vi "is_finished.vi"(8 "error in (no error)":errorcluster, 11 "ImagingModeDL090130Frame in":refnum<class "ImagingModeDL090130Frame.lvclass">=refnum) -> (0 "error out":errorcluster, 2 "finished?":bool[](array[boolean]), 3 "ImagingModeDL090130Frame out":refnum<class "ImagingModeDL090130Frame.lvclass">)   [LabVIEW 2010, in "ImagingModeDL090130Frame.lvclass"]
uses:
  ImagingModeDL090130Frame.lvclass
  ImagingModeDL090130Frame.lvclass/ImagingModeDL090130Frame.ctl
panel:
  # "element 0: is sweep finished?\nelement 1: frame finished?\nelement 2: consecutive scanning done?"
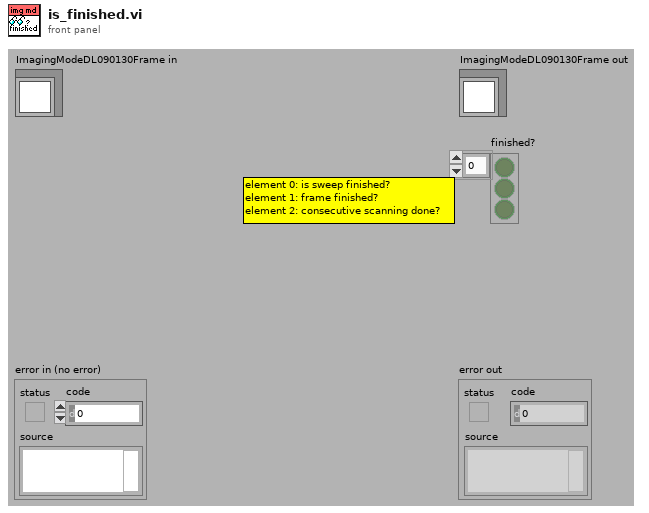
[diagram p1: front panel]
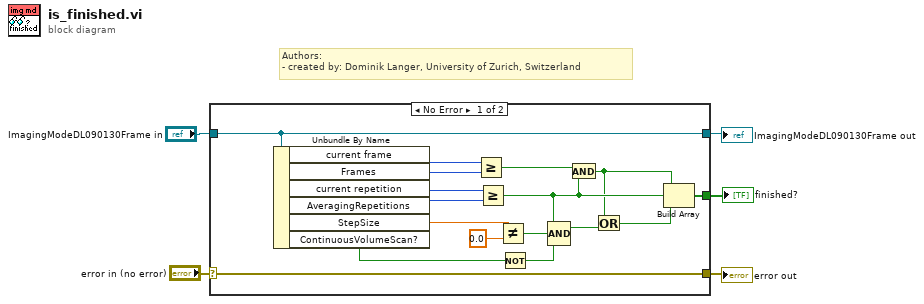
[diagram p0: block diagram]
diagram:
  # "Authors: \n- created by: Dominik Langer, University of Zurich, Switzerland"
  n1 = case shown="No Error" "error in (no error)" {
    selector: "error in (no error)" -> [w13 w24]
    tunnel: [w13 w24] -> w4
    tunnel: [w22 w23] -> w2
    tunnel: "ImagingModeDL090130Frame in" -> [w22 w23]
    tunnel: [w14 _] -> w1
    frame No Error {
      n2 = Unbundle By Name(w22) -> ("current frame"=w21:i32, "Frames"=w20:i32, "current repetition"=w19:i32, "AveragingRepetitions"=w18:i32, "StepSize"=w12:dbl[unit], "ContinuousVolumeScan?"=w8:bool)
      n3 = Greater Or Equal?(x=w21, y=w20) -> (x >= y?=w16:bool)
      n4 = Greater Or Equal?(x=w19, y=w18) -> (x >= y?=w15:bool)
      n5 = Not Equal?(x=w12, y=dbl[unit] 0.0) -> (x != y?=w10:bool)
      n6 = Not(x=w8) -> (.not. x?=w7:bool)
      n7 = Compound Arithmetic op=AND(w15, w10, w7) -> (w17:bool)
      n8 = And(x=w16, y=w15) -> (x .and. y?=w9:bool)
      n9 = Or(x=w9, y=w17) -> (x .or. y?=w6:bool)
      n10 = Build Array(w9, w15, w6) -> (w14:bool[])
    }
    frame Error {
    }
  }
  "error out" <- w4
  "ImagingModeDL090130Frame out" <- w2
  "finished?" <- w1
